vi "Lin_SendData.vi"(4 "Seq?":bool, 5 "NAD":u8 format="%.0x", 6 "Data":T2=[{"send?"=TRUE, "payload"=[2, 16, 3, 255, 255, 255, 255, 255], "Delays"=100, "Note"="", "mult?"=FALSE, "Seq"=0}] {"payload" format="%02x"}, 7 "mode":enum16{"EntDig", "Send"}(ring)=enum."Send", 8 "Error In":errorcluster caption="错误输入", 11 "LIN Device":T1={"Master Frame(3C)"="MasterReq\nSPA3414_ConfigurationsCMAGeely_CEMCALYPSOSDB34XX0Cfg_LIN3_190709_", "Slave Frame(3D)"="SlaveResp\nSPA3414_ConfigurationsCMAGeely_CEMCALYPSOSDB34XX0Cfg_LIN3_190709_", "Request Schedule"="CEMLIN3DiagRequestSchedule\nSPA3414_ConfigurationsCMAGeely_CEMCALYPSOSDB34XX0Cfg_LIN3_190709_", "Response Schedule"="CEMLIN3DiagResponseSchedule\nSPA3414_ConfigurationsCMAGeely_CEMCALYPSOSDB34XX0Cfg_LIN3_190709_", "Frame Write SCU"="", "Frame Read SCU"="", "LIN Name"=""}) -> (0 "error IO":errorcluster, 3 "LIN Device":T1={"Master Frame(3C)"="MasterReq\nSPA3414_ConfigurationsCMAGeely_CEMCALYPSOSDB34XX0Cfg_LIN3_190709_", "Slave Frame(3D)"="SlaveResp\nSPA3414_ConfigurationsCMAGeely_CEMCALYPSOSDB34XX0Cfg_LIN3_190709_", "Request Schedule"="CEMLIN3DiagRequestSchedule\nSPA3414_ConfigurationsCMAGeely_CEMCALYPSOSDB34XX0Cfg_LIN3_190709_", "Response Schedule"="CEMLIN3DiagResponseSchedule\nSPA3414_ConfigurationsCMAGeely_CEMCALYPSOSDB34XX0Cfg_LIN3_190709_", "Frame Write SCU"="", "Frame Read SCU"="", "LIN Name"=""})   [LabVIEW 2018]
uses:
  Crl/LIN_DataType.ctl
  user VI's/LIN/LIN Device.ctl
panel:
  in  "EntDig":T2=[{"send?"=TRUE, "payload"=[2, 16, 97, 255, 255, 255, 255], "Delays"=100, "Note"="", "mult?"=FALSE, "Seq"=0}, {"send?"=TRUE, "payload"=[2, 39, 97, 255, 255, 255, 255], "Delays"=100, "Note"="", "mult?"=FALSE, "Seq"=0}, {"send?"=TRUE, "payload"=[4, 39, 98, 255, 255, 255, 255], "Delays"=100, "Note"="", "mult?"=FALSE, "Seq"=0}] {"payload" format="%02x"}
  # "ms"
  # "ms"
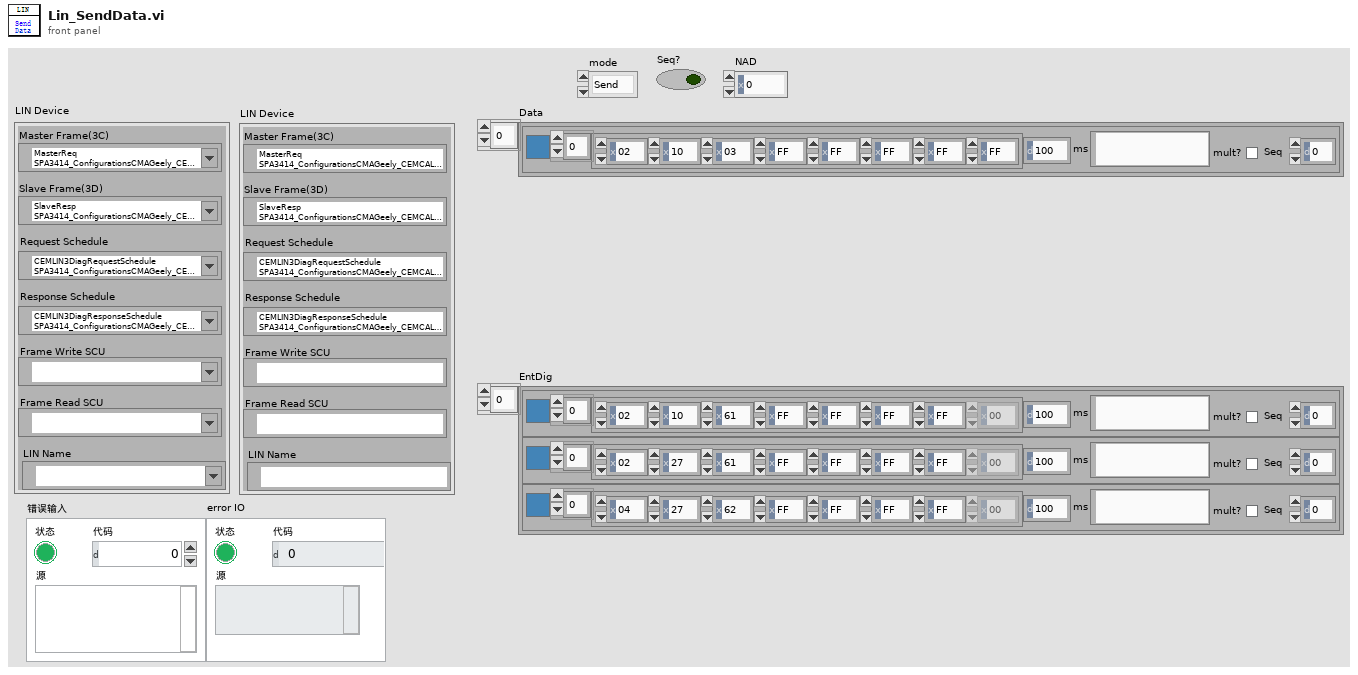
[diagram p1: front panel]
types:
  T1 = typedef "LIN Device.ctl" = cluster{"Master Frame(3C)":refnum<k21>, "Slave Frame(3D)":refnum<k21>, "Request Schedule":refnum<k21>, "Response Schedule":refnum<k21>, "Frame Write SCU":refnum<k21>, "Frame Read SCU":refnum<k21>, "LIN Name":refnum<k21>}
  T2 = typedef "LIN_DataType.ctl" = cluster{"send?":bool, "payload":u8[], "Delays":u32, "Note":string, "mult?":bool, "Seq":i32}[]
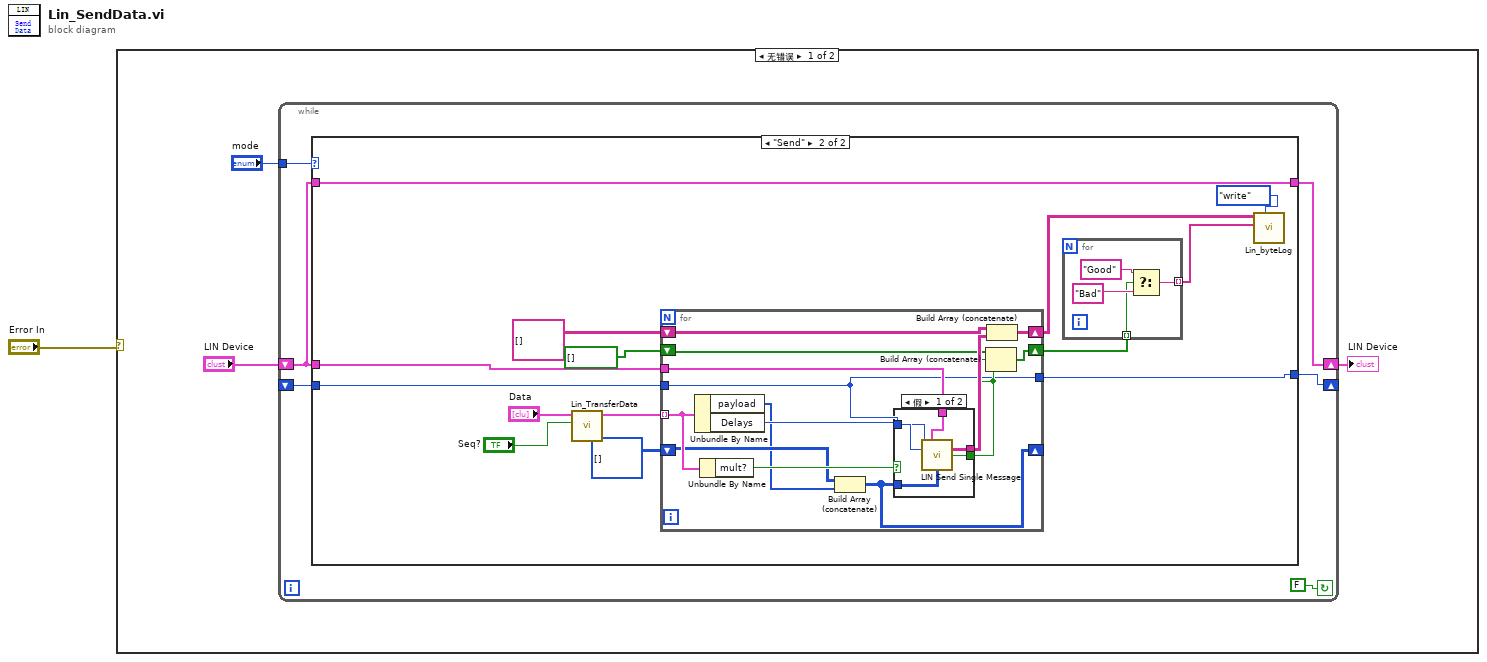
[diagram p0: block diagram]
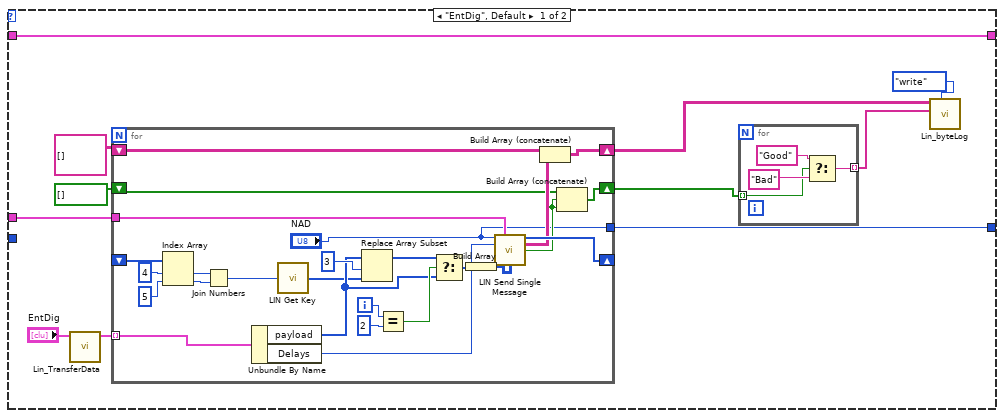
[diagram p2: hidden frame]
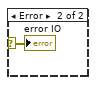
[diagram p4: hidden frame]
diagram:
  n1 = case shown="无错误" "Error In" {
    selector: "Error In" -> [_ w90]
    frame No Error {
      n2 = while {
        tunnel: "mode" -> [w10]
        shift-right: [w7] -> w2
        shift-left: "LIN Device" -> [w8]
        shift-right: [w5] -> _
        shift-left: _ -> [w6]
        stop <- FALSE continue-if-true
        n3 = case shown="\"Send\"" w10 {
          tunnel: w8 -> [w21 w62]
          tunnel: w8 -> [w19 w61]
          tunnel: [w19 w61] -> w7
          tunnel: w6 -> [_ w59]
          tunnel: [w16 w58] -> w5
          frame "EntDig", Default {
            n4 = call "Lin_TransferData.vi"("Data"="EntDig") -> ("Data"=w11:T2)  [unwired: 10 in]
            n5 = for {
              tunnel: w11 -> [w51] mode=indexing
              shift-right: [w38] -> _
              shift-left: _ -> [w43]
              tunnel: w21 -> [w39]
              shift-right: [w30] -> w13
              shift-left: string[][] [] -> [w32]
              shift-right: [w28] -> w12
              shift-left: bool[] [] ("数组") -> [w29]
              tunnel: ["NAD"] -> w16
              i -> [w49]
              n6 = Index Array(array=w43, index #1=4 ("索引"), index #2=5 ("索引")) -> (element #1=w45:u8, element #2=w44:u8)
              n7 = Join Numbers(hi=w45, lo=w44) -> ((hi.lo)=w42:u16)
              n8 = Unbundle By Name(w51) -> ("payload"=w36:u8[], "Delays"=w33:u32)
              n9 = call "LIN Get Key.vi"("x"=w42) -> ("KEY"=w35:u8[])
              n10 = Replace Array Subset(array=w36, new element=w35, index=3 ("索引")) -> (w34:u8[])
              n11 = Equal?(x=w49, y=2) -> (x = y?=w41:bool)
              n12 = Select(t=w34, s=w41, f=w36) -> (s? t:f=w40:u8[])
              n13 = Build Array(w40) -> (w50:u8[][])
              n14 = call "LIN Send Single Message.vi"("NAD"="NAD", "LIN Device"=w39, "Msg Wait T"=w33, "Tx Msg"=w50) -> ("Rx Msg"=w38:u8[], "TxRx Data"=w31:string[][], "Response Good?"=w27:bool)  [unwired: 6 in, 3 out]
              n15 = Build Array (concatenate)(w32, w31) -> (w30:string[][])
              n16 = Build Array (concatenate)(w29, w27, w27) -> (w28:bool[])
            }
            n17 = for {
              tunnel: [w23] -> w15 mode=indexing
              tunnel: w12 -> [w22] mode=indexing
              n18 = Select(t="Good", s=w22, f="Bad") -> (s? t:f=w23:string)
            }
            n19 = call "Lin_byteLog.vi"("r/w"=enum16{"read", "write"}."write", "RespGood?"=w15, "TxRx Data"=w13) -> ()  [unwired: 8 in, 1 out]
          }
          frame "Send" {
            n20 = call "Lin_TransferData.vi"("Seq?"="Seq?", "Data"="Data") -> ("Data"=w64:T2)  [unwired: 9 in]
            n21 = for {
              tunnel: w64 -> [w74] mode=indexing
              tunnel: w62 -> [w83]
              shift-right: [w79] -> w55
              shift-left: string[][] [] -> [w81]
              shift-right: [w78] -> w54
              shift-left: bool[] [] ("数组") -> [w76]
              tunnel: w59 -> [w75]
              tunnel: [w75] -> w58
              shift-right: [w70] -> _
              shift-left: u8[][] [] -> [w72]
              n22 = Unbundle By Name(w74) -> ("payload"=w71:u8[], "Delays"=w82:u32)
              n23 = Unbundle By Name(w74) -> ("mult?"=w73:bool)
              n24 = Build Array (concatenate)(w72, w71) -> (w70:u8[][])
              n25 = case shown="假" w73 {
                tunnel: w83 -> [w89 _]
                tunnel: w82 -> [w88 _]
                tunnel: [w87 _] -> w80
                tunnel: [w86 _] -> w77
                tunnel: w75 -> [w85 _]
                tunnel: w70 -> [w84 _]
                frame False {
                  n26 = call "LIN Send Single Message.vi"("NAD"=w85, "LIN Device"=w89, "Msg Wait T"=w88, "Tx Msg"=w84) -> ("TxRx Data"=w87:string[][], "Response Good?"=w86:bool)  [unwired: 6 in, 4 out]
                }
                frame True {
                }
              }
              n27 = Build Array (concatenate)(w76, w77, w77) -> (w78:bool[])
              n28 = Build Array (concatenate)(w81, w80) -> (w79:string[][])
            }
            n29 = for {
              tunnel: [w67] -> w57 mode=indexing
              tunnel: w54 -> [w66] mode=indexing
              n30 = Select(t="Good", s=w66, f="Bad") -> (s? t:f=w67:string)
            }
            n31 = call "Lin_byteLog.vi"("r/w"=enum16{"read", "write"}."write", "RespGood?"=w57, "TxRx Data"=w55) -> ()  [unwired: 8 in, 1 out]
          }
        }
      }
      "LIN Device" <- w2
    }
    frame Error {
      "error IO" <- w90
    }
  }
